vi "GetZT.vi"(8 "error in (no error)":errorcluster, 11 "connection ID":refnum<k5>) -> (0 "error out":errorcluster, 1 "Theta (rad)":dbl, 2 "Z":dbl, 3 "connection ID out":refnum<k5>)   [LabVIEW 2018]
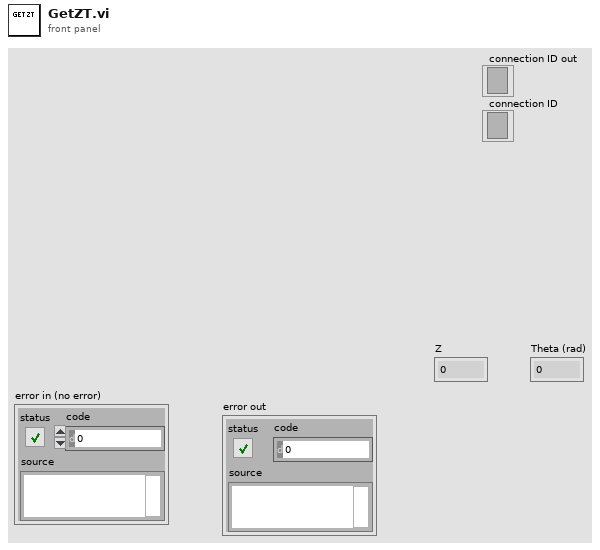
[diagram p1: front panel]
types:
  T1 = enum16{"Standard", "Buffered", "CRLF", "Immediate"}
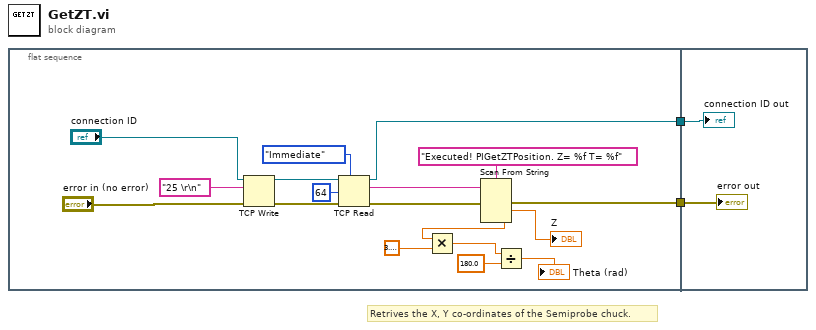
[diagram p0: block diagram]
diagram:
  # "Retrives the X, Y co-ordinates of the Semiprobe chuck."
  n1 = flat-sequence {
    tunnel: [w7] -> w2
    tunnel: [w6] -> w1
    tunnel: w2 -> [w22]
    tunnel: w1 -> [w21]
    frame #0 {
      n2 = TCP Write(connection ID="connection ID", data in="25 \r\n", error in (no error)="error in (no error)") -> (connection ID out=w4:refnum<k5>, error out=w19:errorcluster)  [unwired: 1 in, 1 out]
      n3 = TCP Read(connection ID=w4, bytes to read=64, error in (no error)=w19, 7:T1."Immediate" ("mode (standard)")) -> (connection ID out=w6:refnum<k5>, data out=w18:string, error out=w16:errorcluster)  [unwired: 1 in]
      n4 = Scan From String(format string="Executed! PIGetZTPosition. Z= %f T= %f", input string=w18, error in=w16) -> (error out=w7:errorcluster, output 1=→"Z":dbl, output 2=w12:dbl)  [unwired: 3 in, 2 out]
      n5 = Multiply(x=w12, y=3.141592653589793) -> (x*y=w9:dbl)
      n6 = Divide(x=w9, y=180.0) -> (x/y=→"Theta (rad)":dbl)
    }
    frame #1 {
      "error out" <- w22
      "connection ID out" <- w21
    }
  }
